vi "Experimental Data Save VI Reference.vi"(2 "Input":refnum<vi>, 3 "Action":T1) -> (0 "Output":refnum<vi>)   [LabVIEW 2013]
uses:
  Action.ctl
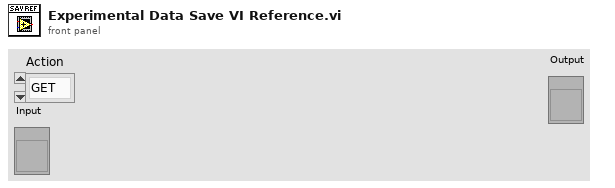
[diagram p1: front panel]
types:
  T1 = typedef "Action.ctl" = enum16{"GET", "PUT", "DELETE"}
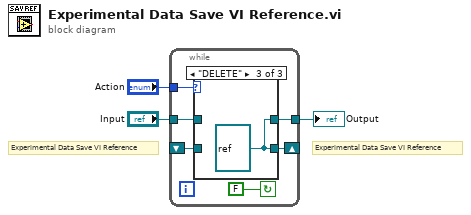
[diagram p0: block diagram]
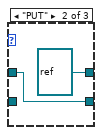
[diagram p3: hidden frame]
diagram:
  # "Experimental Data Save VI Reference"
  # "Experimental Data Save VI Reference"
  n1 = while {
    shift-right: [w6] -> _
    shift-left: _ -> [w5]
    tunnel: "Action" -> [w8]
    tunnel: "Input" -> [w7]
    tunnel: [w4] -> w1
    stop <- FALSE continue-if-true
    n2 = case shown="\"DELETE\"" w8 {
      tunnel: w7 -> [_ w12 _]
      tunnel: [w10 w12 w13] -> w6
      tunnel: w5 -> [w10 _ _]
      tunnel: [w10 refnum<vi> refnum ("Input") w13] -> w4
      frame "GET", Default {
      }
      frame "PUT" {
      }
      frame "DELETE" {
        w13 = refnum<vi> refnum ("Input")
      }
    }
  }
  "Output" <- w1
